vi "Global 1.vi"() -> ()   [LabVIEW 2014]
uses:
  Control 1.ctl
panel:
  in  "Forklift Out":bool
  in  "Forklift In":T1
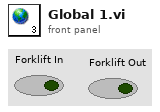
[diagram p1: front panel]
types:
  T1 = typedef "Control 1.ctl" = bool
diagram:
